vi "Create IMAQ references.vi"(8 "error in (no error)":errorcluster, 11 "Retiga in":refnum<class "Retiga.lvclass">) -> (0 "error out":errorcluster, 3 "Retiga out":refnum<class "Retiga.lvclass">)   [LabVIEW 2012, in "Retiga.lvclass"]
uses:
  Retiga.lvclass
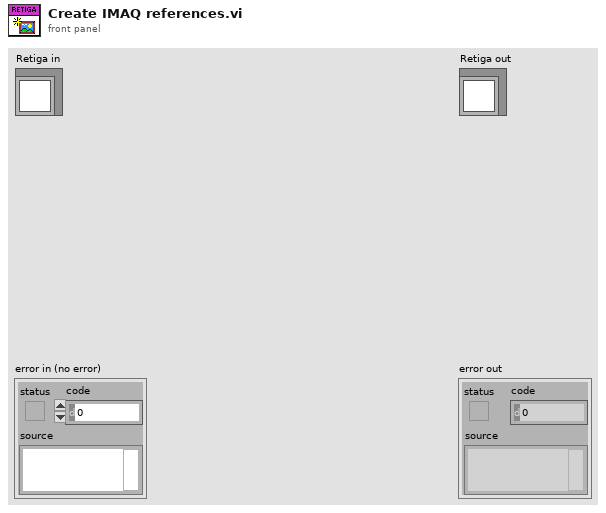
[diagram p1: front panel]
types:
  T1 = typedef "Image Type" = u32
  T2 = typedef "IMAQ Image.ctl" = refnum<image>
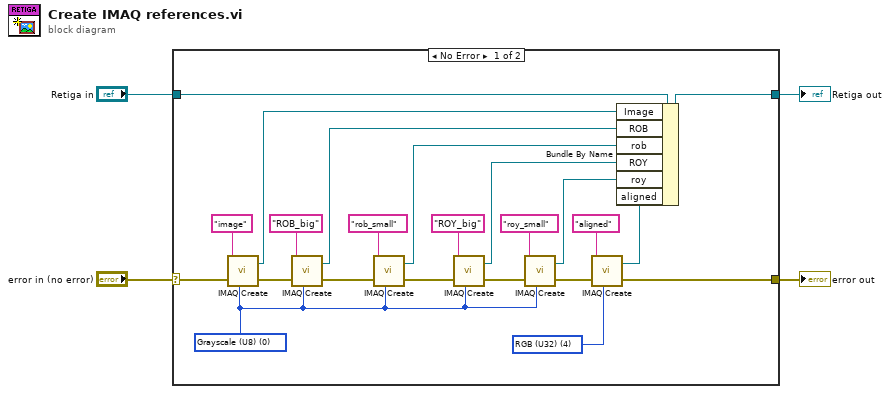
[diagram p0: block diagram]
diagram:
  n1 = case shown="No Error" "error in (no error)" {
    selector: "error in (no error)" -> [w20 w29]
    tunnel: [w19 w29] -> w3
    tunnel: [w26 w28] -> w1
    tunnel: "Retiga in" -> [w27 w28]
    frame No Error {
      w17 = T1 4 items=["Grayscale (U8)", "Grayscale (I16)", "Grayscale (SGL)", "Complex (CSG)", "RGB (U32)", "HSL (U32)", "RGB (U64)", "Grayscale (U16)"] ("Image Type")
      w18 = T1 0 items=["Grayscale (U8)", "Grayscale (I16)", "Grayscale (SGL)", "Complex (CSG)", "RGB (U32)", "HSL (U32)", "RGB (U64)", "Grayscale (U16)"] ("Image Type")
      n2 = call "IMAQ Create"("Image Name"="image", "Image Type"=w18, "error in (no error)"=w20) -> ("New Image"=w10:T2, "error out"=w25:errorcluster)  [unwired: 2 in]
      n3 = call "IMAQ Create"("Image Name"="ROB_big", "Image Type"=w18, "error in (no error)"=w25) -> ("New Image"=w9:T2, "error out"=w24:errorcluster)  [unwired: 2 in]
      n4 = call "IMAQ Create"("Image Name"="rob_small", "Image Type"=w18, "error in (no error)"=w24) -> ("New Image"=w8:T2, "error out"=w23:errorcluster)  [unwired: 2 in]
      n5 = call "IMAQ Create"("Image Name"="ROY_big", "Image Type"=w18, "error in (no error)"=w23) -> ("New Image"=w7:T2, "error out"=w22:errorcluster)  [unwired: 2 in]
      n6 = call "IMAQ Create"("Image Name"="roy_small", "Image Type"=w18, "error in (no error)"=w22) -> ("New Image"=w6:T2, "error out"=w21:errorcluster)  [unwired: 2 in]
      n7 = call "IMAQ Create"("Image Name"="aligned", "Image Type"=w17, "error in (no error)"=w21) -> ("New Image"=w5:T2, "error out"=w19:errorcluster)  [unwired: 2 in]
      n8 = Bundle By Name(cluster=w27, "Image"=w10, "ROB"=w9, "rob"=w8, "ROY"=w7, "roy"=w6, "aligned"=w5) -> (w26:refnum<class "Retiga.lvclass">)
    }
    frame Error {
    }
  }
  "error out" <- w3
  "Retiga out" <- w1
